vi "Create.vi"(0 "reference in":refnum<class "Simulated-PowerModule.lvclass">, 5 "configuration":string, 11 "Error In":errorcluster) -> (4 "reference out":refnum<class "Simulated-PowerModule.lvclass">, 6 "ProcessVI Ref":refnum<vi>, 15 "Error Out":errorcluster)   [LabVIEW 2023, in "Simulated-PowerModule.lvlib" / "Simulated-PowerModule.lvclass"]
uses:
  Simulated-PowerModule.lvclass
  Configuration.ctl
  builds/PowerModuleInterface/PowerModuleInterface.lvlibp/Classes/PowerModule_interface/Range.ctl
  builds/PowerModuleInterface/PowerModuleInterface.lvlibp/Classes/PowerModule_interface/Limits.ctl
  builds/PowerModuleInterface/PowerModuleInterface.lvlibp/Classes/PowerModule_interface/Measurements.ctl
  Simulated-PowerModule.lvclass/Simulated-PowerModule.ctl
  <vilib>/addons/_JKI.lib/Serialization/JSON/JKI JSON Serialization.lvlib
  <vilib>/Utility/LVLibp/NI_PackedLibraryUtility.lvlib
  builds/PowerModuleInterface/PowerModuleInterface.lvlibp/Classes/PowerModule_interface/PowerModuleInterface.lvclass
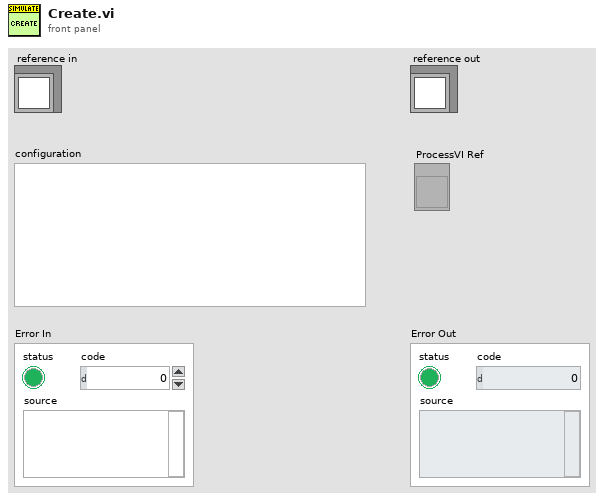
[diagram p1: front panel]
types:
  T1 = enum32{"invalid app kind", "Development System", "Run Time System", "Student Edition", "Embedded LabVIEW", "Evaluation", "Custom"}
  T2 = typedef "PowerModuleInterface.lvlibp/PowerModuleInterface.lvclass/Measurements.ctl" = cluster{"measured voltage (V)":dbl, "measured current (A)":dbl, "setpoint voltage (V)":dbl, "setpoint current (A)":dbl, "timestamp":dbl}
  T3 = enum16{"open", "replace", "create", "open or create", "replace or create", "replace or create with confirmation"}
  T4 = typedef "Simulated-PowerModule.lvlib/Simulated-PowerModule.lvclass/Configuration.ctl" = cluster{"range":T5, "Limits":T6}
  T5 = typedef "PowerModuleInterface.lvlibp/PowerModuleInterface.lvclass/Range.ctl" = cluster{"Current Max (A)":dbl, "Current Min (A)":dbl, "Voltage Max (V)":dbl, "Voltage Min (V)":dbl}
  T6 = typedef "PowerModuleInterface.lvlibp/PowerModuleInterface.lvclass/Limits.ctl" = cluster{"Current Max (A)":dbl, "Current Min (A)":dbl, "Voltage Max (V)":dbl, "Voltage Min (V)":dbl, "Power Max (W)":dbl, "Power Min (W)":dbl}
  T7 = typedef "Simulated-PowerModule.lvlib/Simulated-PowerModule.lvclass/ObjectAttributes.ctl" = cluster{"JSON Config Path":path, "mode":T8, "Configuration":T4, "connected":bool, "reserved":bool, "energized":bool, "output enabled":bool, "setpoint":cluster{"voltage":dbl, "current":dbl, "resistance":dbl}, "last timestamp":i64, "measurement array":T2[], "profile":dbl[][], "step dt":i64, "measurement array size":u32}
  T8 = typedef "Simulated-PowerModule.lvlib/Simulated-PowerModule.lvclass/Mode.ctl" = u16
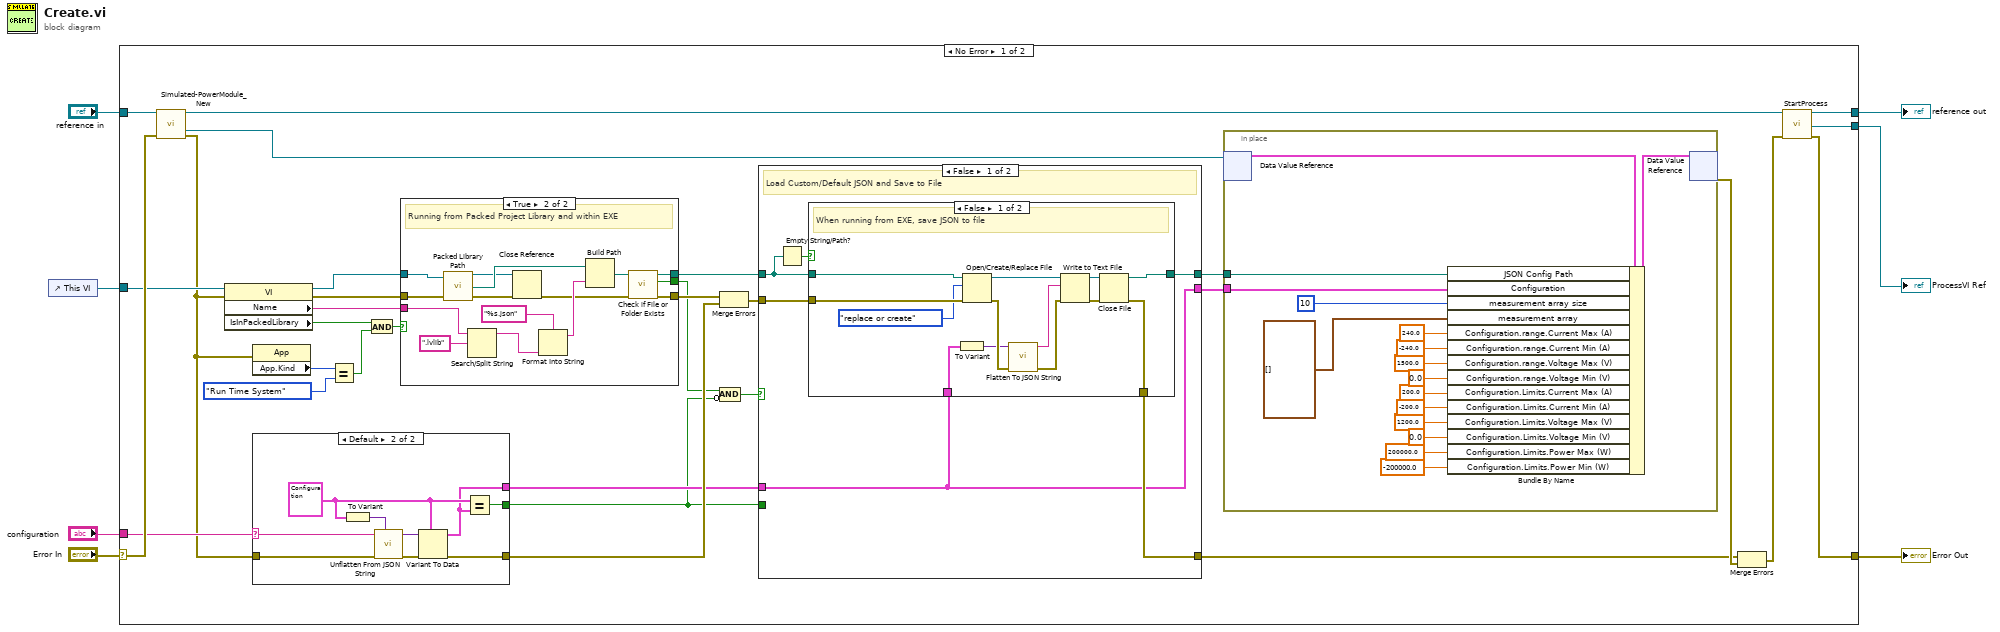
[diagram p0: block diagram]
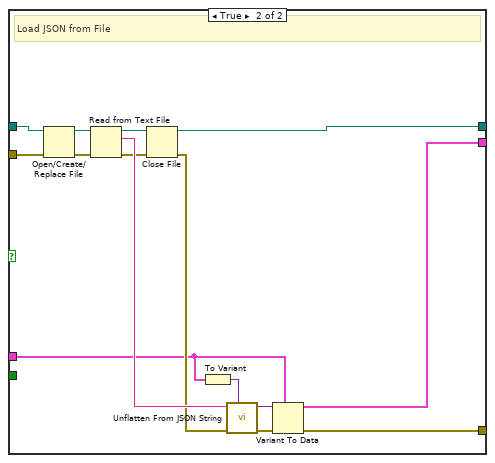
[diagram p3: hidden frame]
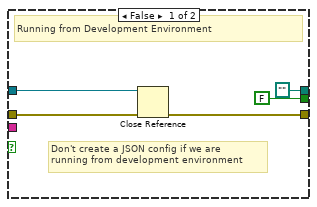
[diagram p4: hidden frame]
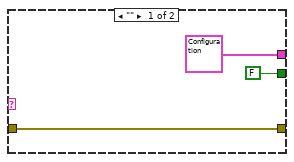
[diagram p5: hidden frame]
diagram:
  n1 = control-ref of="This VI"() -> (w1:refnum<vi>)
  n2 = case shown="No Error" "Error In" {
    selector: "Error In" -> [w37 w123]
    tunnel: "reference in" -> [w38 w124]
    tunnel: "configuration" -> [w29 _]
    tunnel: [w34 w124] -> w4
    tunnel: [w31 w123] -> w3
    tunnel: [w30 _] -> w2
    tunnel: w1 -> [w28 _]
    frame No Error {
      n3 = call "Simulated-PowerModule_New.vi"("reference in"=w38, "Error In"=w37) -> ("reference out"=w35:refnum<class "Simulated-PowerModule.lvclass">, "DVRRefOut"=w36:refnum<data-value>, "Error Out"=w13:errorcluster)  [unwired: 10 in, 1 out]
      n4 = property class="VI"(reference=w28, error in=w13) -> (reference out=w26:refnum<vi>, error out=w27:errorcluster, "Name"=w14:string, "IsInPackedLibrary"=w10:bool)
      n5 = property class="App"(error in=w13) -> ("App.Kind"=w12:T1)  [unwired: 1 in, 2 out]
      n6 = case shown="Default" w29 {
        selector: w29 -> [_ w119]
        tunnel: w13 -> [w113 w122]
        tunnel: [T4 {"range"={"Current Max (A)"=61557.0, "Current Min (A)"=61557.0, "Voltage Max (V)"=0.0, "Voltage Min (V)"=5000.0}, "Limits"={"Current Max (A)"=0.0, "Current Min (A)"=0.0, "Voltage Max (V)"=0.0, "Voltage Min (V)"=0.0, "Power Max (W)"=0.0, "Power Min (W)"=0.0}} ("Configuration") w116] -> w19
        tunnel: [FALSE w115] -> w18
        tunnel: [w113 w114] -> w24
        frame "" {
        }
        frame Default {
          w117 = T4 {"range"={"Current Max (A)"=61557.0, "Current Min (A)"=61557.0, "Voltage Max (V)"=0.0, "Voltage Min (V)"=5000.0}, "Limits"={"Current Max (A)"=0.0, "Current Min (A)"=0.0, "Voltage Max (V)"=0.0, "Voltage Min (V)"=0.0, "Power Max (W)"=0.0, "Power Min (W)"=0.0}} ("Configuration")
          n7 = To Variant(anything=w117) -> (Variant=w120:variant)
          n8 = call <vilib>:"Unflatten From JSON String.vi"("Type and Defaults"=w120, "error in"=w122, "JSON String"=w119) -> ("error out"=w121:errorcluster, "Variant"=w118:variant)  [unwired: 7 in]
          n9 = Variant To Data(error in=w121, type=w117, Variant=w118) -> (data=w116:T4, error out=w114:errorcluster)
          n10 = Equal?(x=w117, y=w116) -> (x = y?=w115:bool)
        }
      }
      n11 = Equal?(x=w12, y=T1."Run Time System") -> (x = y?=w9:bool)
      n12 = And(x=w10, y=w9) -> (x .and. y?=w8:bool)
      n13 = case shown="True" w8 {
        tunnel: w27 -> [w94 w110]
        tunnel: w26 -> [w93 w109]
        tunnel: [w92 w102] -> w25
        tunnel: [FALSE ("file or folder exists?") w101] -> w22
        tunnel: [path "" w100] -> w20
        tunnel: w14 -> [_ w99]
        frame False {
          # "Don't create a JSON config if we are \nrunning from development environment"
          # "Running from Development Environment"
          n14 = Close Reference(reference=w93, error in (no error)=w94) -> (error out=w92:errorcluster)
        }
        frame True {
          # "Running from Packed Project Library and within EXE"
          n15 = call <vilib>:"Packed Library Path.vi"("error in (no error)"=w110, "vi reference"=w109) -> ("error out"=w98:errorcluster, "packed library path"=w105:path, "vi reference out"=w97:refnum<vi>)  [unwired: 1 in]
          n16 = Search/Split String(string=w99, search string/char (-)=".lvlib") -> (substring before match=w107:string)  [unwired: 1 in, 2 out]
          n17 = Close Reference(reference=w97, error in (no error)=w98) -> (error out=w96:errorcluster)
          n18 = Format Into String(format string="%s.json", w107) -> (resulting string=w104:string)  [unwired: 2 in, 1 out]
          n19 = Build Path(base path=w105, name or relative path=w104) -> (appended path=w103:path)
          n20 = call <vilib>:"Check if File or Folder Exists.vi"("error in (no error)"=w96, "path"=w103) -> ("error out"=w102:errorcluster, "file or folder exists?"=w101:bool, "dup path"=w100:path)  [unwired: 7 in]
        }
      }
      n21 = Merge Errors(w25, w24) -> (w23:errorcluster)
      n22 = Compound Arithmetic op=AND(w22, invert w18) -> (w21:bool)
      n23 = case shown="False" w21 {
        tunnel: w23 -> [w60 w90]
        tunnel: w20 -> [w58 w89]
        tunnel: w19 -> [w55 w79]
        tunnel: w18 -> [_ _]
        tunnel: [w55 w77] -> w17
        tunnel: [w59 w78] -> w16
        tunnel: [w56 w76] -> w15
        frame False {
          # "Load Custom/Default JSON and Save to File"
          n24 = Empty String/Path?(string/path=w58) -> (empty?=w57:bool)
          n25 = case shown="False" w57 {
            tunnel: w60 -> [w70 w75]
            tunnel: [w68 w75] -> w59
            tunnel: w55 -> [w64 _]
            tunnel: w58 -> [w62 w74]
            tunnel: [w61 w74] -> w56
            frame False {
              # "When running from EXE, save JSON to file"
              n26 = To Variant(anything=w64) -> (Variant=w63:variant)
              n27 = Open/Create/Replace File(file path (use dialog)=w62, error in=w70, operation (0:open)=T3."replace or create") -> (refnum out=w73:refnum<file>, error out=w66:errorcluster)  [unwired: 3 in, 1 out]
              n28 = call <vilib>:"Flatten To JSON String.vi"("error in"=w66, "Variant"=w63) -> ("error out"=w67:errorcluster, "JSON String"=w65:string)  [unwired: 8 in]
              n29 = Write to Text File(file (use dialog)=w73, text=w65, error in=w67) -> (refnum out=w71:refnum<file>, error out=w72:errorcluster)  [unwired: 1 in, 1 out]
              n30 = Close File(refnum=w71, error in=w72) -> (path=w61:path, error out=w68:errorcluster)
            }
            frame True {
              # "Don't save to file when running from dev environment"
            }
          }
        }
        frame True {
          # "Load JSON from File"
          n31 = Open/Create/Replace File(file path (use dialog)=w89, error in=w90) -> (refnum out=w87:refnum<file>, error out=w88:errorcluster)  [unwired: 4 in, 1 out]
          n32 = Read from Text File(file (use dialog)=w87, error in=w88) -> (refnum out=w83:refnum<file>, text=w86:string, error out=w84:errorcluster)  [unwired: 2 in, 1 out]
          n33 = Close File(refnum=w83, error in=w84) -> (path=w76:path, error out=w82:errorcluster)
          n34 = To Variant(anything=w79) -> (Variant=w85:variant)
          n35 = call <vilib>:"Unflatten From JSON String.vi"("Type and Defaults"=w85, "error in"=w82, "JSON String"=w86) -> ("error out"=w81:errorcluster, "Variant"=w80:variant)  [unwired: 7 in]
          n36 = Variant To Data(error in=w81, type=w79, Variant=w80) -> (data=w77:T4, error out=w78:errorcluster)
        }
      }
      n37 = in-place {
        in-place-border: w17 -> [w51]
        in-place-border: w15 -> [w52]
        n38 = in-place-dvr #1(w36) -> (w53:T7)  [unwired: 1 out]
        n39 = Bundle By Name(cluster=w53, "JSON Config Path"=w52, "Configuration"=w51, "measurement array size"=u32 10, "measurement array"=T2[] [], "Configuration.range.Current Max (A)"=240.0, "Configuration.range.Current Min (A)"=-240.0, "Configuration.range.Voltage Max (V)"=1500.0, "Configuration.range.Voltage Min (V)"=0.0, "Configuration.Limits.Current Max (A)"=200.0, "Configuration.Limits.Current Min (A)"=-200.0, "Configuration.Limits.Voltage Max (V)"=1200.0, "Configuration.Limits.Voltage Min (V)"=0.0, "Configuration.Limits.Power Max (W)"=200000.0, "Configuration.Limits.Power Min (W)"=-200000.0 ("Configuration.Limits.Power Max (W)")) -> (w54:T7)
        n40 = in-place-dvr #1(w54) -> (w33:errorcluster)  [unwired: 1 out]
      }
      n41 = Merge Errors(w16, w33) -> (w32:errorcluster)
      n42 = call "StartProcess.vi"("reference in"=w35, "Error In"=w32) -> ("reference out"=w34:refnum<class "Simulated-PowerModule.lvclass">, "ProcessViRef"=w30:refnum<vi>, "Error Out"=w31:errorcluster)  [unwired: 13 in, 2 out]
    }
    frame Error {
    }
  }
  "Error Out" <- w3
  "reference out" <- w4
  "ProcessVI Ref" <- w2
